vi "U64 to I32.vi"(2 "error in (no error)":errorcluster, 3 "U64":dbl) -> (0 "error out":errorcluster, 1 "I32":i32)   [LabVIEW 2017]
panel:
  # "LVHDF5 Toolkit\nCopyright (c) 2005-2013 by Jason D. Sommerville\nCopyright (c) 2014 by UPVI, LLC.\n\nThis use and distribution of this file is governed by the terms found in \nLICENSE.txt distributed with this toolkit and installed at\n <user.lib>\\_lvhdf5\\LICENSE.txt"
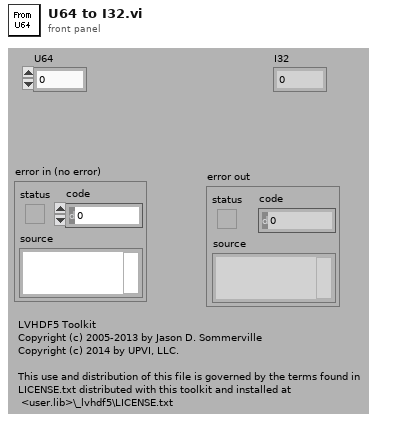
[diagram p1: front panel]
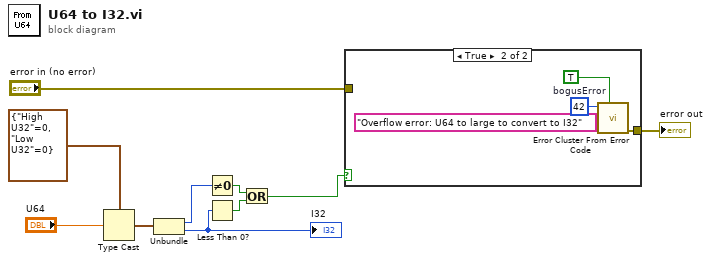
[diagram p0: block diagram]
diagram:
  n1 = Type Cast(type=cluster{"High U32":u32, "Low U32":i32} {"High U32"=0, "Low U32"=0}, x="U64") -> (*(type *) &x=w8:cluster{"High U32":u32, "Low U32":i32})
  n2 = Unbundle(w8) -> ("High U32"=w4:u32, "Low U32"=w5:i32)
  "I32" <- w5
  n3 = Not Equal To 0?(x=w4) -> (x != 0?=w3:bool)
  n4 = Less Than 0?(x=w5) -> (x < 0?=w2:bool)
  n5 = Or(x=w3, y=w2) -> (x .or. y?=w1:bool)
  n6 = case shown="True" w1 {
    tunnel: [w11 w12] -> w7
    tunnel: "error in (no error)" -> [w11 _]
    frame False {
    }
    frame True {
      w15 = 42  # bogusError
      n7 = call <vilib>:"Error Cluster From Error Code.vi"("show call chain? (False)"=TRUE, "error message (\"\")"="Overflow error: U64 to large to convert to I32" ("error message (\"\")"), "error code (0)"=w15) -> ("error out"=w12:errorcluster)  [unwired: 6 in]
    }
  }
  "error out" <- w7
